vi "FL Map Interval.vi"(8 "x1":dbl, 9 "x0":dbl, 10 "b":dbl, 11 "a":dbl) -> (2 "m":dbl, 3 "k":dbl)   [LabVIEW 2017, in "NI_Fuzzy_Logic_API.lvlib"]
uses:
  <vilib>/addons/Fuzzy Logic/NI_Fuzzy_Logic_API.lvlib
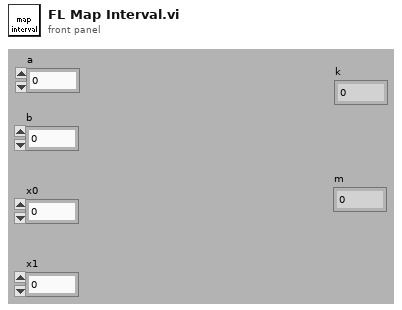
[diagram p1: front panel]
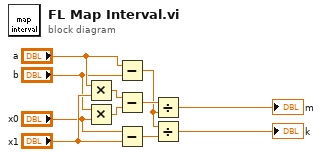
[diagram p0: block diagram]
diagram:
  n1 = Multiply(x="a", y="x1") -> (x*y=w7:dbl)
  n2 = Multiply(x="b", y="x0") -> (x*y=w6:dbl)
  n3 = Subtract(x="a", y="b") -> (x-y=w3:dbl)
  n4 = Subtract(x=w7, y=w6) -> (x-y=w5:dbl)
  n5 = Subtract(x="x0", y="x1") -> (x-y=w4:dbl)
  n6 = Divide(x=w5, y=w3) -> (x/y=→"m":dbl)
  n7 = Divide(x=w3, y=w4) -> (x/y=→"k":dbl)
